vi "Display.vi"(8 "error in":errorcluster, 11 "Timeout Two Button in":refnum<class "Timeout Two Button.lvclass">) -> (0 "error out":errorcluster, 3 "Timeout Two Button out":refnum<class "Timeout Two Button.lvclass">)   [LabVIEW 2021, in "Pop-Up.lvlib" / "Timeout Two Button.lvclass"]
doc: "This vi displays the two button timeout popup.\n\n<b>Code Developed By:</b> +\nDaniel Coons +\nhttps://github.com/danielcoons/tsc-pop-up"
uses:
  Timeout Two Button.lvclass
  C:/Development/Open Source/tsc-pop-up/Popup/Popup.lvclass
  Timeout Two Button.lvclass/Timeout Two Button.ctl
  Popup/Popup.lvclass/Popup.ctl
  Popup/Data Member Access/Read Theme.vi
  Theme/Theme.lvclass
  Popup/Popup.lvclass
  user32.dll
panel:
  out "count":string
  in  "n-choice":bool
  in  "y-choice":bool
  out "header":bool
  out "2D Picture":picture
  out "String":string
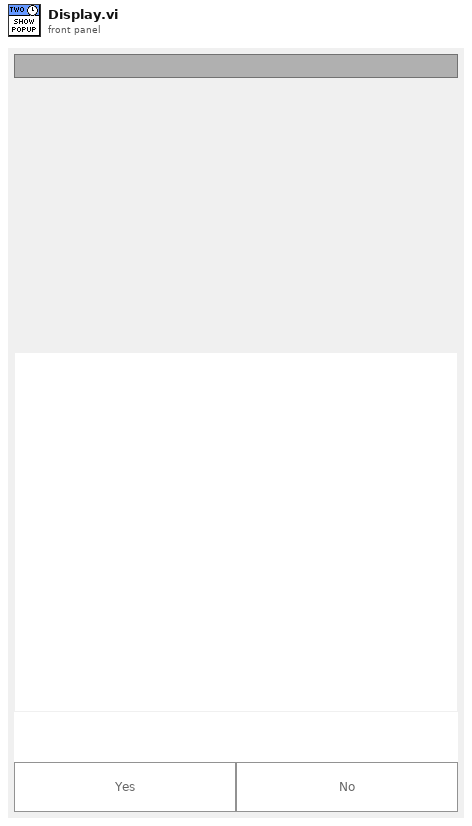
[diagram p1: front panel]
types:
  T1 = typedef "LVPoint32TypeDef.ctl" = cluster{"Horizontal":i32, "Vertical":i32}
  T2 = typedef "LVPositionTypeDef.ctl" = cluster{"Left":i32, "Top":i32}
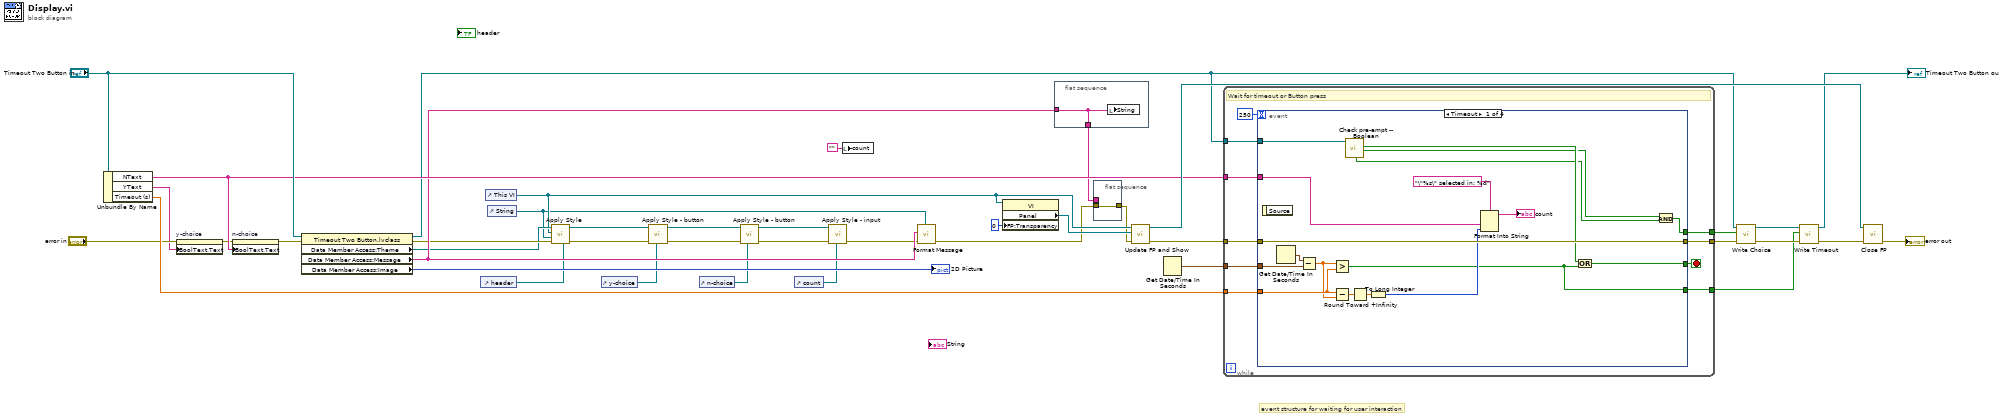
[diagram p0: block diagram]
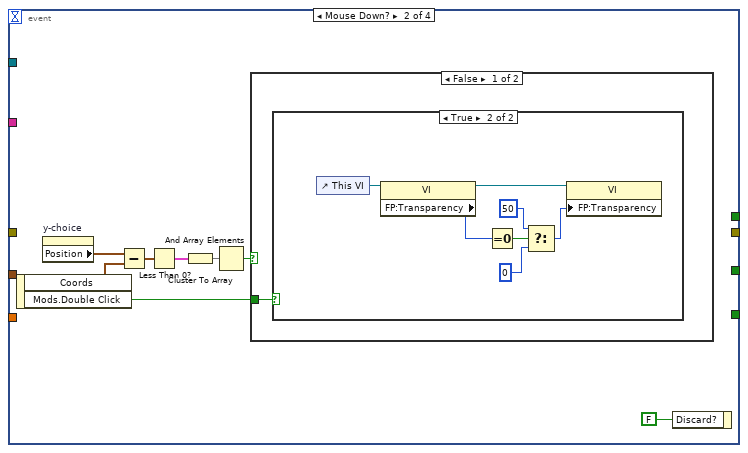
[diagram p2: hidden frame]
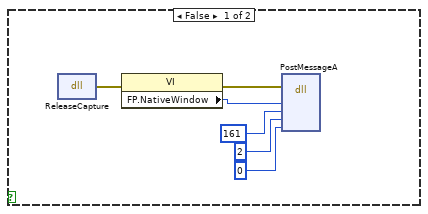
[diagram p3: hidden frame]
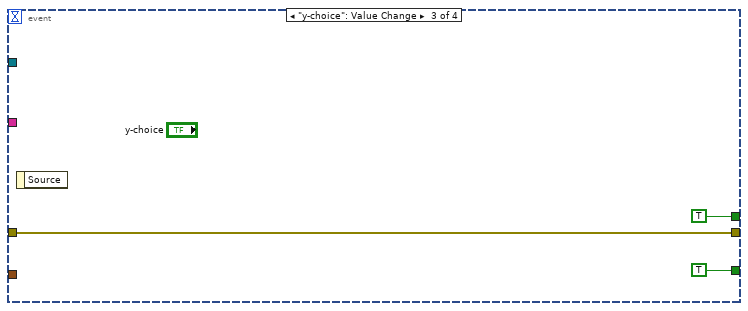
[diagram p5: hidden frame]
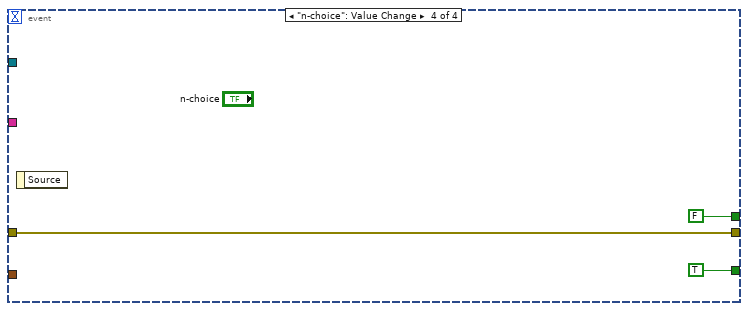
[diagram p6: hidden frame]
diagram:
  # "event structure for waiting for user interaction"
  n1 = Unbundle By Name("Timeout Two Button in") -> ("NText"=w31:string, "YText"=w28:string, "Timeout (s)"=w39:dbl)
  n2 = property on="y-choice" class="Bool"(error in="error in", "BoolText.Text"=w28) -> (error out=w30:errorcluster)  [unwired: 1 in, 1 out]
  n3 = property on="n-choice" class="Bool"(error in=w30, "BoolText.Text"=w31) -> (error out=w32:errorcluster)  [unwired: 1 in, 1 out]
  n4 = property class="Timeout Two Button.lvclass"(reference="Timeout Two Button in", error in=w32) -> (reference out=w27:refnum<class "Timeout Two Button.lvclass">, error out=w24:errorcluster, "Data Member Access:Theme"=w23:refnum<class "Theme.lvclass">, "Data Member Access:Message"=w26:string, "Data Member Access:Image"=→"2D Picture":picture)
  n5 = control-ref of="header"() -> (w21:refnum<vi>)
  n6 = control-ref of="This VI"() -> (w20:refnum<vi>)
  n7 = control-ref of="String"() -> (w19:refnum<vi>)
  n8 = call "Apply Style.vi"("header ref"=w21, "error in"=w24, "message ref"=w19, "pop up ref"=w20, "Theme in"=w23) -> ("error out"=w22:errorcluster, "Theme out"=w17:refnum<class "Theme.lvclass">)  [unwired: 5 in]
  n9 = control-ref of="y-choice"() -> (w16:refnum<vi>)
  n10 = call "Apply Style - button.vi"("button ref"=w16, "error in"=w22, "Theme in"=w17) -> ("error out"=w18:errorcluster, "Theme out"=w14:refnum<class "Theme.lvclass">)  [unwired: 7 in]
  n11 = control-ref of="n-choice"() -> (w13:refnum<vi>)
  n12 = call "Apply Style - button.vi"("button ref"=w13, "error in"=w18, "Theme in"=w14) -> ("error out"=w15:errorcluster, "Theme out"=w11:refnum<class "Theme.lvclass">)  [unwired: 7 in]
  n13 = control-ref of="count"() -> (w10:refnum<vi>)
  n14 = call "Apply Style - input.vi"("input ref"=w10, "error in (no error)"=w15, "Theme in"=w11) -> ("error out"=w12:errorcluster)  [unwired: 7 in, 1 out]
  n15 = local write "count"("" ("count")) -> ()
  n16 = call "Format Message.vi"("formatted string"=w19, "error in"=w12, "String Input"=w26) -> ("error out"=w3:errorcluster)  [unwired: 7 in, 1 out]
  n17 = property class="VI"(reference=w20, "FP:Transparency"=u8 0 ("Front Panel Window:Transparency")) -> ("Panel"=w36:refnum<vi>)  [unwired: 1 in, 2 out]
  n18 = flat-sequence {
    tunnel: w26 -> [w43]
    tunnel: [w43] -> w1
    frame #0 {
      n19 = local write "String"(w43) -> ()
    }
  }
  n20 = flat-sequence {
    tunnel: w3 -> [w44]
    tunnel: [w44] -> w2
    tunnel: w1 -> [_]
    frame #0 {
    }
  }
  n21 = call "Update FP and Show.vi"("error in (no error)"=w2, "Panel Ref"=w36, "VI in"=w20) -> ("error out"=w35:errorcluster, "VI out"=w33:refnum<vi>)  [unwired: 7 in]
  n22 = Get Date/Time In Seconds() -> (seconds since 1Jan1904=w40:timestamp)
  n23 = while {
    tunnel: w35 -> [w50]
    tunnel: [w49] -> w38
    tunnel: w40 -> [w54]
    tunnel: w39 -> [w52]
    tunnel: [w48] -> w37
    tunnel: w31 -> [w47]
    tunnel: w27 -> [w46]
    tunnel: [w45] -> w4
    stop <- w53 stop-if-true
    # "Wait for timeout or Button press"
    n24 = event shown="[0] Timeout" {
      selector: _ -> [_ _ _ _]
      dyn-events: _ -> [_ _ _ _]
      timeout: 250 -> [_ _ _ _]
      tunnel: w54 -> [w71 _ _ _]
      tunnel: [w65 _ TRUE TRUE] -> w53
      tunnel: w52 -> [w70 _ _ _]
      tunnel: w50 -> [w67 _ w97 w100]
      tunnel: [w67 _ w97 w100] -> w49
      tunnel: [w62 _ TRUE FALSE] -> w48
      tunnel: w47 -> [w59 _ _ _]
      tunnel: w46 -> [w64 _ _ _]
      tunnel: [w55 _ _ _] -> w45
      event Timeout {
        n25 = event-data() -> ()  [unwired: 1 in, 1 out]
        n26 = Get Date/Time In Seconds() -> (seconds since 1Jan1904=w72:timestamp)
        n27 = Subtract(x=w72, y=w71) -> (x-y=w69:dbl)
        n28 = Greater?(x=w69, y=w70) -> (0:w55:bool)
        n29 = Subtract(x=w70, y=w69) -> (x-y=w68:dbl)
        n30 = call "Check pre-empt -- Boolean.vi"("_Popup in"=w64) -> ("Value?"=w61:bool, "Pre-empted?"=w63:bool, "Type Match?"=w60:bool)  [unwired: 7 in, 1 out]
        n31 = Round Toward +Infinity(x=w68) -> (ceil(x): smallest int >= x=w57:dbl)
        n32 = To Long Integer(number=w57) -> (32bit integer=w58:i32)
        n33 = Format Into String(format string="\"%s\" selected in: %d", w59, w58) -> (resulting string=→"count":string)  [unwired: 2 in, 1 out]
        n34 = Or(x=w63, y=w55) -> (x .or. y?=w65:bool)
        n35 = And(x=w61, y=w60) -> (x .and. y?=w62:bool)
      }
      event Mouse Down? {
        n36 = event-data() -> ("Coords"=w75:T1, "Mods.Double Click"=w73:bool)  [unwired: 1 in]
        n37 = property on="y-choice" class="Bool"() -> ("Position"=w79:T2)  [unwired: 2 in, 2 out]
        n38 = Subtract(x=w79, y=w75) -> (x-y=w78:T2)
        n39 = Less Than 0?(x=w78) -> (x < 0?=w77:cluster{"Left":bool, "Top":bool})
        n40 = Cluster To Array(cluster=w77) -> (array=w76:bool[])
        n41 = And Array Elements(Boolean array=w76) -> (logical AND=w74:bool)
        n42 = case shown="False" w74 {
          tunnel: w73 -> [w81 _]
          frame False {
            n43 = case shown="True" w81 {
              frame False {
                n44 = dll-call lib="user32.dll" fn="ReleaseCapture"() -> (error out=w85:errorcluster)  [unwired: 4 in, 1 out]
                n45 = property class="VI"(error in=w85) -> (error out=w86:errorcluster, "FP.NativeWindow"=w87:u64)  [unwired: 1 in, 1 out]
                n46 = dll-call lib="user32.dll" fn="PostMessageA"(error in=w86, "hWnd"=w87, "Msg"=161, "wParam"=2, "lParam"=0) -> ()  [unwired: 7 in, 2 out]
              }
              frame True {
                n47 = control-ref of="This VI"() -> (w94:refnum<vi>)
                n48 = property class="VI"(reference=w94) -> (reference out=w92:refnum<vi>, "FP:Transparency"=w93:u8)  [unwired: 1 in, 1 out]
                n49 = Equal To 0?(x=w93) -> (x = 0?=w91:bool)
                n50 = Select(t=u8 50, s=w91, f=u8 0) -> (s? t:f=w90:u8)
                n51 = property class="VI"(reference=w92, "FP:Transparency"=w90) -> ()  [unwired: 1 in, 2 out]
              }
            }
          }
          frame True {
          }
        }
        n52 = event-data("Discard?"=FALSE) -> ()  [unwired: 1 in, 1 out]
      }
      event "y-choice": Value Change {
        n53 = event-data() -> ()  [unwired: 1 in, 1 out]
      }
      event "n-choice": Value Change {
        n54 = event-data() -> ()  [unwired: 1 in, 1 out]
      }
    }
  }
  n55 = call-dynamic "Write Choice.vi"("error in (no error)"=w38, "Choice"=w37, "_Popup in"=w27) -> ("error out"=w42:errorcluster, "_Popup out"=w6:refnum<class "Timeout Two Button.lvclass">)  [unwired: 7 in]
  n56 = call "Write Timeout.vi"("error in"=w42, "Timeout?"=w4, "Popup in"=w6) -> ("error out"=w7:errorcluster, "Popup out"=→"Timeout Two Button out":refnum<class "Timeout Two Button.lvclass">)  [unwired: 7 in]
  n57 = call "Close FP.vi"("error in (no error)"=w7, "VI in"=w33) -> ("error out"=→"error out":errorcluster)  [unwired: 9 in]
